vi "close_ser.vi"(0 "error in":errorcluster, 1 "VISA resource name in":refnum<visa-resource-name>) -> ()   [LabVIEW 2009]
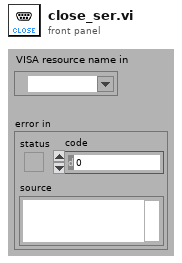
[diagram p1: front panel]
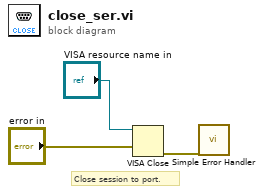
[diagram p0: block diagram]
diagram:
  # "Close session to port."
  n1 = VISA Close(VISA resource name="VISA resource name in", error in (no error)="error in") -> (error out=w3:errorcluster)
  n2 = call <vilib>:"Simple Error Handler.vi"("error in (no error)"=w3) -> ()  [unwired: 1 in, 8 out]
